vi "CVT Enum IndexRead.vi"(3 "error in (no error)":errorcluster, 5 "Tag Index":i32) -> (0 "error out":errorcluster, 1 "Value":i32)   [LabVIEW 2014, in "QwaveSys Raspberry Pi Library.lvlib"]
uses:
  QwaveSys Raspberry Pi Library.lvlib
  _SubVIs/TypeDefs/cvt_MemBlock Methods.ctl
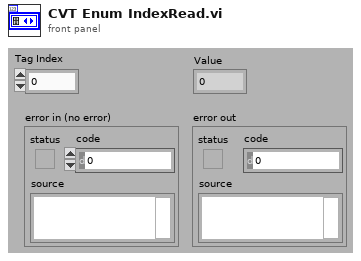
[diagram p1: front panel]
types:
  T1 = typedef "QwaveSys Raspberry Pi Library.lvlib/cvt_MemBlock Methods.ctl" = enum16{"init", "read", "readall", "write"}
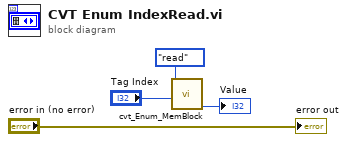
[diagram p0: block diagram]
diagram:
  n1 = call "cvt_Enum_MemBlock.vi"("Index"="Tag Index", "Method"=cvt_MemBlock_Methods."read") -> ("Value"=→"Value":i32)  [unwired: 2 in, 7 out]
  "error out" <- "error in (no error)"
